vi "Find Top and Error Terminals.vi"(7 "Position":T1, 8 "error in (no error)":errorcluster, 11 "Array":refnum<vi>[](array[refnum])) -> (0 "error out":errorcluster, 2 "Error out":refnum<vi>, 3 "Top out":refnum<vi>)   [LabVIEW 2016]
uses:
  <resource>/dialog/QuickDrop/plugins/_WireMultipleSupport/Connector Pane Position.ctl
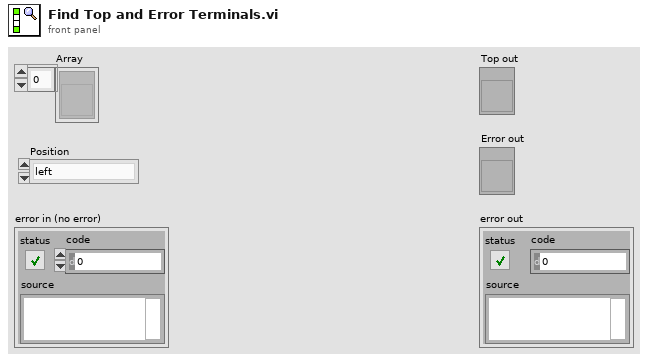
[diagram p1: front panel]
types:
  T1 = typedef "Connector Pane Position.ctl" = enum16{"left", "right"}
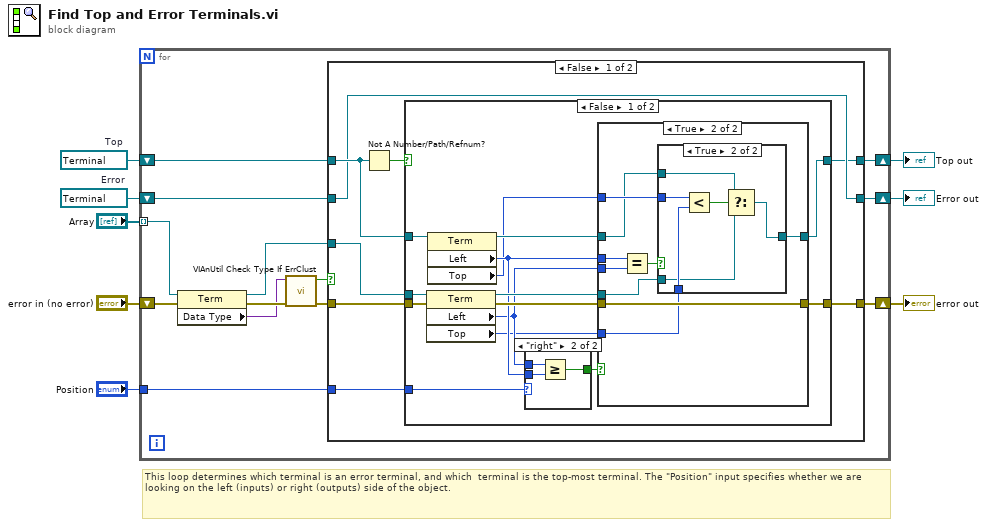
[diagram p0: block diagram]
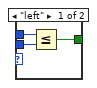
[diagram p2: hidden frame]
diagram:
  w6 = refnum<vi> refnum  # Error
  w3 = refnum<vi> refnum  # Top
  # "This loop determines which terminal is an error terminal, and which  terminal is the top-most terminal. The \"Position\" input specifies whether we are looking on the left (inputs) or right (outputs) side of the object."
  n1 = for {
    shift-right: [w12] -> w8
    shift-left: "error in (no error)" -> [w21]
    shift-right: [w10] -> w5
    shift-left: w3 -> [w14]
    tunnel: "Array" -> [w20] mode=indexing
    shift-right: [w11] -> w7
    shift-left: w6 -> [w15]
    tunnel: "Position" -> [w9]
    n2 = property class="Term"(reference=w20, error in=w21) -> (reference out=w13:refnum<vi>, error out=w19:errorcluster, "Data Type"=w18:variant)
    n3 = call <vilib>:"VIAnUtil Check Type If ErrClust.vi"("error in (no error)"=w19, "Data In"=w18) -> ("error out"=w17:errorcluster, "IsErrClust?"=w16:bool)  [unwired: 8 out]
    n4 = case shown="False" w16 {
      tunnel: w17 -> [w29 w72]
      tunnel: w15 -> [w24 _]
      tunnel: w14 -> [w26 w70]
      tunnel: w13 -> [w28 w71]
      tunnel: [w27 w72] -> w12
      tunnel: [w24 w71] -> w11
      tunnel: [w23 w70] -> w10
      tunnel: w9 -> [w22 _]
      frame False {
        n5 = Not A Number/Path/Refnum?(number/path/refnum=w26) -> (NaN/Path/Refnum?=w25:bool)
        n6 = case shown="False" w25 {
          tunnel: w29 -> [w43 w69]
          tunnel: w28 -> [w42 w68]
          tunnel: [w37 w69] -> w27
          tunnel: w26 -> [w36 _]
          tunnel: [w35 w68] -> w23
          tunnel: w22 -> [w30 _]
          frame False {
            n7 = property class="Term"(reference=w42, error in=w43) -> (reference out=w40:refnum<vi>, error out=w38:errorcluster, "Left"=w33:i32, "Top"=w31:i32)
            n8 = property class="Term"(reference=w36) -> (reference out=w39:refnum<vi>, "Left"=w34:i32, "Top"=w32:i32)  [unwired: 1 in, 1 out]
            n9 = case shown="\"right\"" w30 {
              tunnel: [w44 w49] -> w41
              tunnel: w34 -> [w46 w48]
              tunnel: w33 -> [w45 w47]
              frame "left" {
                n10 = Less Or Equal?(x=w45, y=w46) -> (x <= y?=w44:bool)
              }
              frame "right" {
                n11 = Greater Or Equal?(x=w47, y=w48) -> (x >= y?=w49:bool)
              }
            }
            n12 = case shown="True" w41 {
              tunnel: w40 -> [_ w56]
              tunnel: w39 -> [w50 w52]
              tunnel: w38 -> [w51 w58]
              tunnel: [w51 w58] -> w37
              tunnel: [w50 w55] -> w35
              tunnel: w34 -> [_ w59]
              tunnel: w33 -> [_ w60]
              tunnel: w32 -> [_ w54]
              tunnel: w31 -> [_ w53]
              frame False {
              }
              frame True {
                n13 = Equal?(x=w59, y=w60) -> (x = y?=w57:bool)
                n14 = case shown="True" w57 {
                  tunnel: w56 -> [w61 w63]
                  tunnel: [w61 w62] -> w55
                  tunnel: w54 -> [_ w67]
                  tunnel: w53 -> [_ w66]
                  tunnel: w52 -> [_ w64]
                  frame False {
                  }
                  frame True {
                    n15 = Less?(x=w67, y=w66) -> (x < y?=w65:bool)
                    n16 = Select(t=w64, s=w65, f=w63) -> (s? t:f=w62:refnum<vi>)
                  }
                }
              }
            }
          }
          frame True {
          }
        }
      }
      frame True {
      }
    }
  }
  "error out" <- w8
  "Error out" <- w7
  "Top out" <- w5
